vi "Driver Station Control Data.vi"() -> (0 "Control Data":T1)   [LabVIEW 2012, in "femtoRoboLib.lvlib"]
doc: "Return a cluster containing the control data for the Driver Station (DS). This includes: \n\n<b>Test Mode</b>: True if DS is in Test mode\n<b>FMS Attached</b>: True if connected to the Field Management System\n<b>Autonomous</b>: True if in Autonomous mode\n<b>Enabled</b>: True if enabled\n<b>E-Stopped</b>: True if Emergency Stopped"
uses:
  femtoRoboLib.lvlib
  <vilib>/Rock Robotics/WPI/DriverStation/WPI_DriverStationCommDataCacheOp.ctl
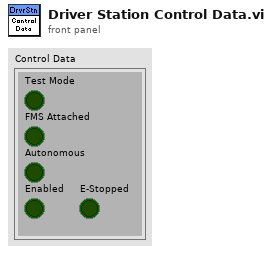
[diagram p1: front panel]
types:
  T1 = cluster{"Test Mode":bool, "FMS Attached":bool, "Autonomous":bool, "Enabled":bool, "E-Stopped":bool}
  T2 = typedef "WPI_DriverStationCommDataCacheOp.ctl" = enum16{"Get", "Set", "Init"}
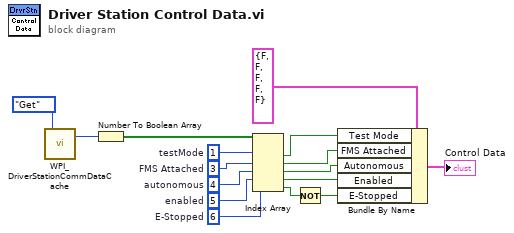
[diagram p0: block diagram]
diagram:
  w9 = 6  # E-Stopped
  w13 = 1  # testMode
  w12 = 3  # FMS Attached
  w11 = 4  # autonomous
  w10 = 5  # enabled
  n1 = call <vilib>:"WPI_DriverStationCommDataCache.vi"("CommDataCacheOp"=WPI_DriverStationCommDataCacheOp."Get") -> ("ControlBit out"=w16:u8)  [unwired: 18 out]
  n2 = Number To Boolean Array(number=w16) -> (Boolean array=w15:bool[])
  n3 = Index Array(array=w15, index #1=w13, index #2=w12, index #3=w11, index #4=w10, index #5=w9) -> (element #1=w6:bool, element #2=w5:bool, element #3=w4:bool, element #4=w3:bool, element #5=w2:bool)
  n4 = Not(x=w2) -> (.not. x?=w1:bool)
  n5 = Bundle By Name(cluster=T1 {"Test Mode"=FALSE, "FMS Attached"=FALSE, "Autonomous"=FALSE, "Enabled"=FALSE, "E-Stopped"=FALSE} ("Cluster"), "Test Mode"=w6, "FMS Attached"=w5, "Autonomous"=w4, "Enabled"=w3, "E-Stopped"=w1) -> (→"Control Data":T1)
